vi "Destroy.vi"(0 "reference in":refnum<class "bodpod.lvclass">, 5 "error in (no error)":errorcluster) -> (14 "reference out":refnum<class "bodpod.lvclass">, 19 "error out":errorcluster)   [LabVIEW 2016, in "bodpod.lvclass"]
doc: "Destructor."
uses:
  bodpod.lvclass
  <vilib>/addons/_AddQ/G#Object/G#Object.lvclass
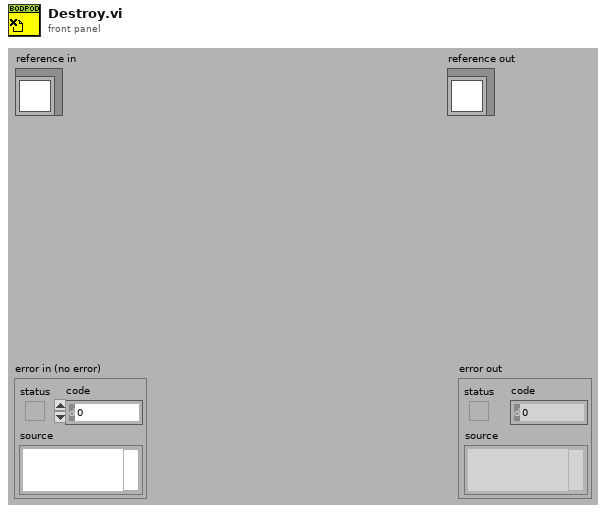
[diagram p1: front panel]
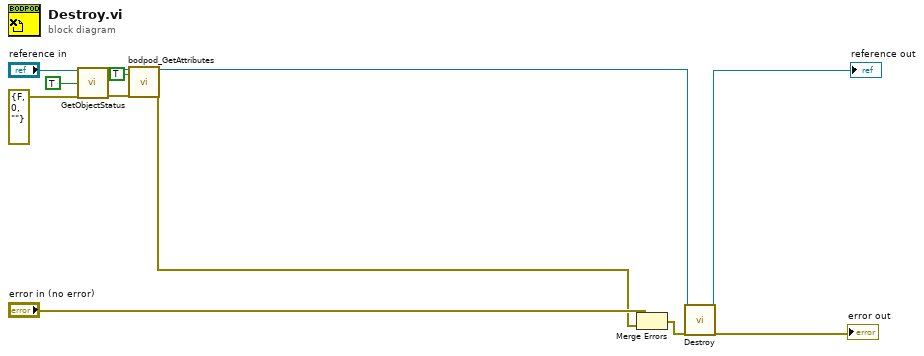
[diagram p0: block diagram]
diagram:
  n1 = call-dynamic "GetObjectStatus.vi"("reference in"="reference in", "simple info (F)"=TRUE ("simple info"), "error in (no error)"=errorcluster {"status"=FALSE, "code"=0, "source"=""}) -> ("reference out"=w5:refnum<class "bodpod.lvclass">, "error out"=w6:errorcluster)  [unwired: 5 in, 10 out]
  n2 = call "bodpod_GetAttributes.vi"("reference in"=w5, "return data? (T)"=TRUE, "error in (no error)"=w6) -> ("reference out"=w4:refnum<class "bodpod.lvclass">, "error out"=w7:errorcluster)  [unwired: 13 in, 2 out]
  n3 = Merge Errors("error in (no error)", w7) -> (w11:errorcluster)
  n4 = call-parent "Destroy.vi"("reference in"=w4, "error in (no error)"=w11) -> ("reference out"=→"reference out":refnum<class "bodpod.lvclass">, "error out"=→"error out":errorcluster)  [unwired: 16 in]
